vi "SpindexerPositionToRotations.vi"(4 "Position (Raw Sensor Units)":i32) -> (1 "Numeric":dbl)   [LabVIEW 2019]
panel:
  in  "gear ratio":dbl=35.0 format="%#_13g"
  in  "resolution":i32=4096
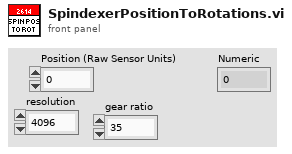
[diagram p1: front panel]
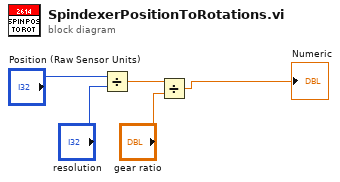
[diagram p0: block diagram]
diagram:
  n1 = Divide(x="Position (Raw Sensor Units)", y="resolution") -> (x/y=w3:dbl)
  n2 = Divide(x=w3, y="gear ratio") -> (x/y=→"Numeric":dbl)
